vi "Add to Tree.vi"(8 "error in (no error)":errorcluster, 9 "Parent Tag":string, 10 "Tree Manager in":refnum<class "Tree Manager.lvclass">, 11 "Data Item in":refnum<class "Data Item.lvclass">) -> (0 "error out":errorcluster, 2 "Tree Manager out":refnum<class "Tree Manager.lvclass">, 3 "Data Item out":refnum<class "Data Item.lvclass">)   [LabVIEW 2023, in "VILab.lvlib" / "Data Item.lvclass"]
uses:
  Data Item.lvclass
  Tree Manager.lvclass
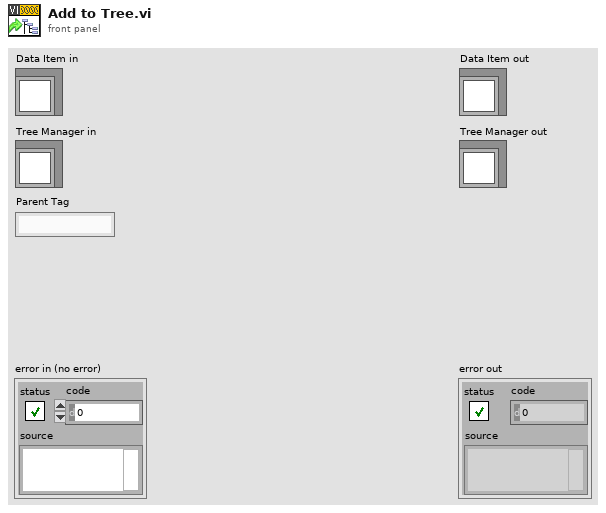
[diagram p1: front panel]
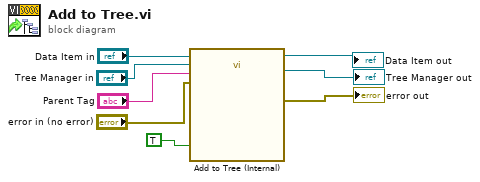
[diagram p0: block diagram]
diagram:
  n1 = call "Add to Tree (Internal).vi"("Add children? (F)"=TRUE, "error in (no error)"="error in (no error)", "Parent Tag"="Parent Tag", "Tree Manager in"="Tree Manager in", "Data Item in"="Data Item in") -> ("error out"=→"error out":errorcluster, "Tree Manager out"=→"Tree Manager out":refnum<class "Tree Manager.lvclass">, "Data Item out"=→"Data Item out":refnum<class "Data Item.lvclass">)  [unwired: 3 in, 1 out]
